vi "Set Updated.vi"(8 "error in (no error)":errorcluster, 10 "Updated":timestamp, 11 "ViaApp in":refnum<class "ViaApp.lvclass">) -> (0 "error out":errorcluster, 3 "ViaApp out":refnum<class "ViaApp.lvclass">)   [LabVIEW 2020, in "PicoG-App.lvlib" / "ViaApp.lvclass"]
uses:
  ViaApp.lvclass
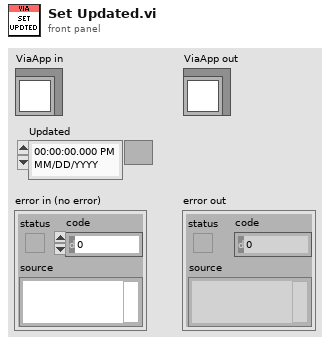
[diagram p1: front panel]
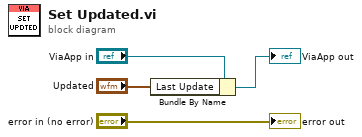
[diagram p0: block diagram]
diagram:
  n1 = Bundle By Name(cluster="ViaApp in", "Last Update"="Updated") -> (→"ViaApp out":refnum<class "ViaApp.lvclass">)
  "error out" <- "error in (no error)"
